vi "niRFUtil FTW Compute Good FFT Size.vi"(0 "Desired FFT Size":i32=1024) -> (4 "Good FFT Size":i32=1024, 6 "FFT Padding":dbl format="%.2f")   [LabVIEW 2015, in "niRFUtil.lvlib"]
uses:
  niRFUtil.lvlib
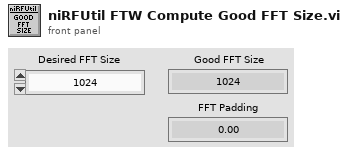
[diagram p1: front panel]
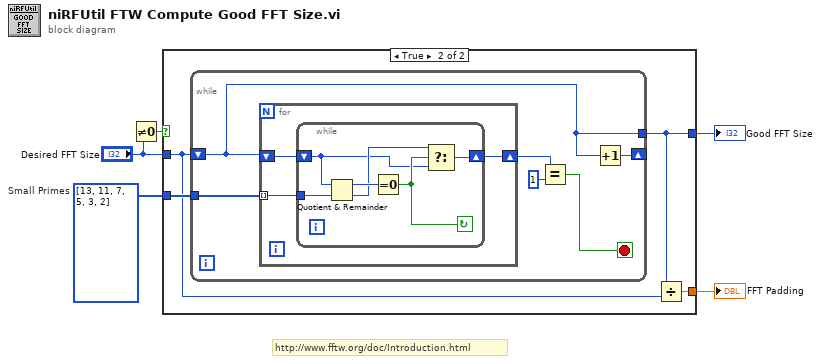
[diagram p0: block diagram]
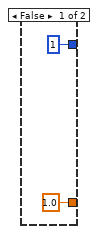
[diagram p2: hidden frame]
diagram:
  w5 = i32[] [13, 11, 7, 5, 3, 2]  # Small Primes
  # "http://www.fftw.org/doc/Introduction.html"
  n1 = Not Equal To 0?(x="Desired FFT Size") -> (x != 0?=w1:bool)
  n2 = case shown="True" w1 {
    tunnel: w5 -> [_ w11]
    tunnel: [1 ("Desired FFT Size") w10] -> w4
    tunnel: [1.0 w9] -> w3
    tunnel: "Desired FFT Size" -> [_ w8]
    frame False {
    }
    frame True {
      n3 = while {
        tunnel: [w12] -> w10
        tunnel: w11 -> [w17]
        shift-left: w8 -> [w12]
        shift-right: [w13] -> _
        stop <- w15 stop-if-true
        n4 = for {
          tunnel: w17 -> [w20] mode=indexing
          shift-right: [w18] -> w14
          shift-left: w12 -> [w19]
          n5 = while {
            shift-left: w19 -> [w22]
            shift-right: [w25] -> w18
            tunnel: w20 -> [w21]
            stop <- w24 continue-if-true
            n6 = Quotient & Remainder(x=w22, y=w21) -> (x-y*floor(x/y)=w26:i32, floor(x/y)=w23:i32)
            n7 = Equal To 0?(x=w26) -> (x = 0?=w24:bool)
            n8 = Select(t=w23, s=w24, f=w22) -> (s? t:f=w25:i32)
          }
        }
        n9 = Equal?(x=w14, y=1) -> (x = y?=w15:bool)
        n10 = Increment(x=w12) -> (x+1=w13:i32)
      }
      n11 = Divide(x=w10, y=w8) -> (x/y=w9:dbl)
    }
  }
  "Good FFT Size" <- w4
  "FFT Padding" <- w3
